vi "UpdatePlugins.vi"(7 "rngInst":refnum<vi>, 8 "Error In Array":errorcluster[](array[cluster]), 10 "Instrument Modules":T1=[{"PluginSelection"=1, "ConfigDialog"=FALSE}, {"PluginSelection"=11, "ConfigDialog"=FALSE}] {"PluginSelection" items=["C37.118 PMU", "C37.118 Sim", "Base PMU", "none", "SiemensDEM0", "AcPwrBase", "Chroma0", "Chroma1", "Chroma2", "NHRDC0", "NHRRGS0", "PPS0"]}, 11 "Current Paths":path[](array[path])) -> (0 "Error Out Array":errorcluster[](array[cluster]), 3 "Current Paths":string[](array[string])=["..\\UserFiles\\Plugins\\AcPwr", "..\\UserFiles\\Plugins\\Sensor"], 4 "PluginTypes":string[](array[string]))   [LabVIEW 2018]
doc: "This VI allows the user to update which Plugins can be selected at the application layer by modifing the location(s) of the INI file(s)."
uses:
  Framework/InstrumentModulesControl.ctl
  <userlib>/NIST/NISTErrorLib/NISTErrorLib.lvlib
panel:
  in  "Save Button":bool
  in  "Update Plugins":bool
  in  "Instrument Modules":T1=[{"PluginSelection"=4, "ConfigDialog"=FALSE}] {"PluginSelection" items=["C37.118 PMU", "C37.118 Sim", "Base PMU", "none", "SiemensDEM0", "AcPwrBase", "Chroma0", "Chroma1", "Chroma2", "NHRDC0", "NHRRGS0", "PPS0"]}
  in  "Cancel  Button":bool
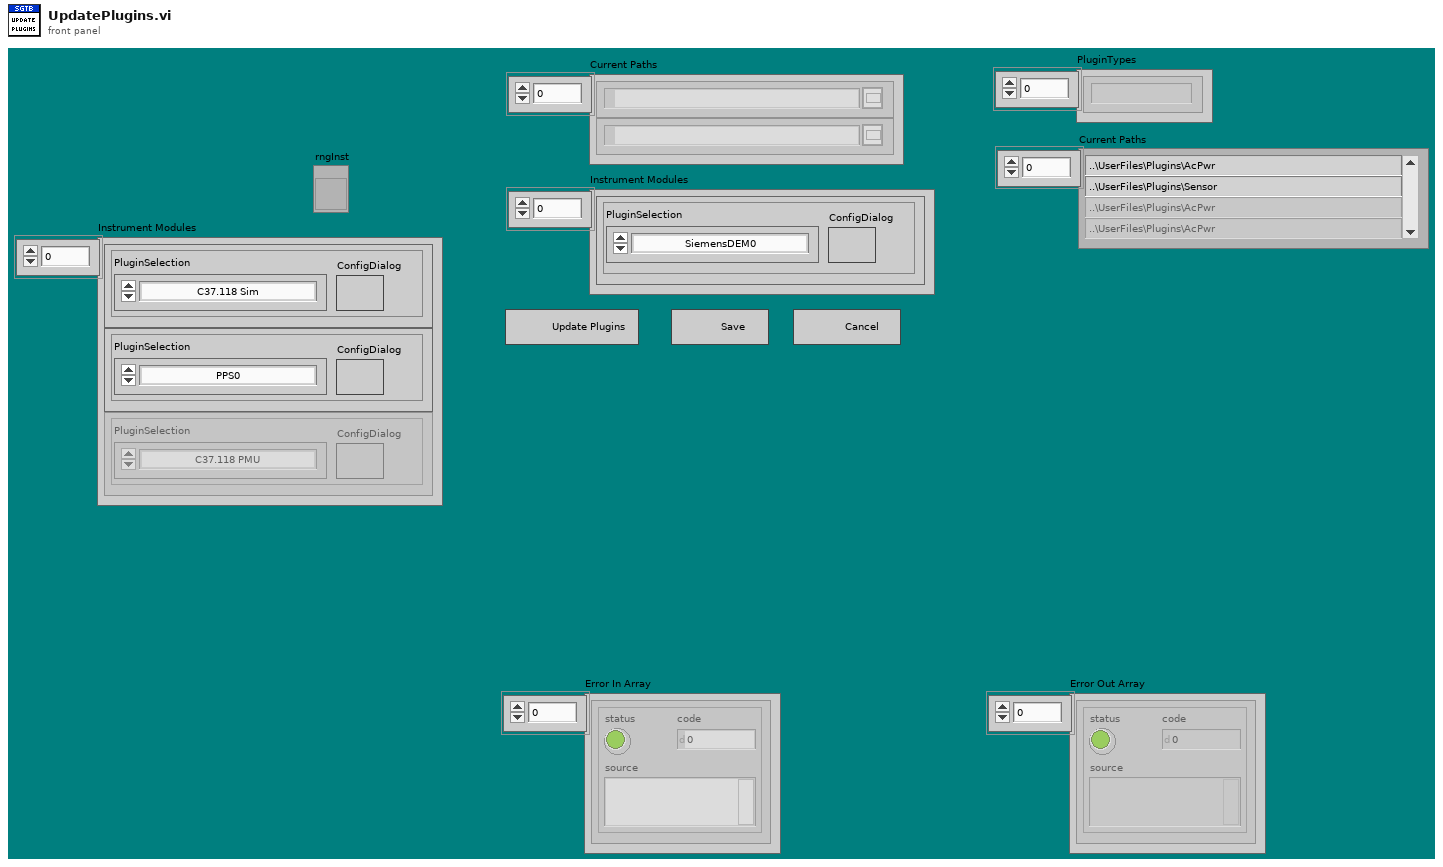
[diagram p1: front panel]
types:
  T1 = typedef "InstrumentModulesControl.ctl" = cluster{"PluginSelection":u16, "ConfigDialog":bool}[]
  T2 = enum32{"Invalid", "Standard", "Closed", "Hidden", "Minimized", "Maximized"}
  T3 = enum32{"Invalid", "Default", "Floating", "Floating/Auto-Hide", "Modal"}
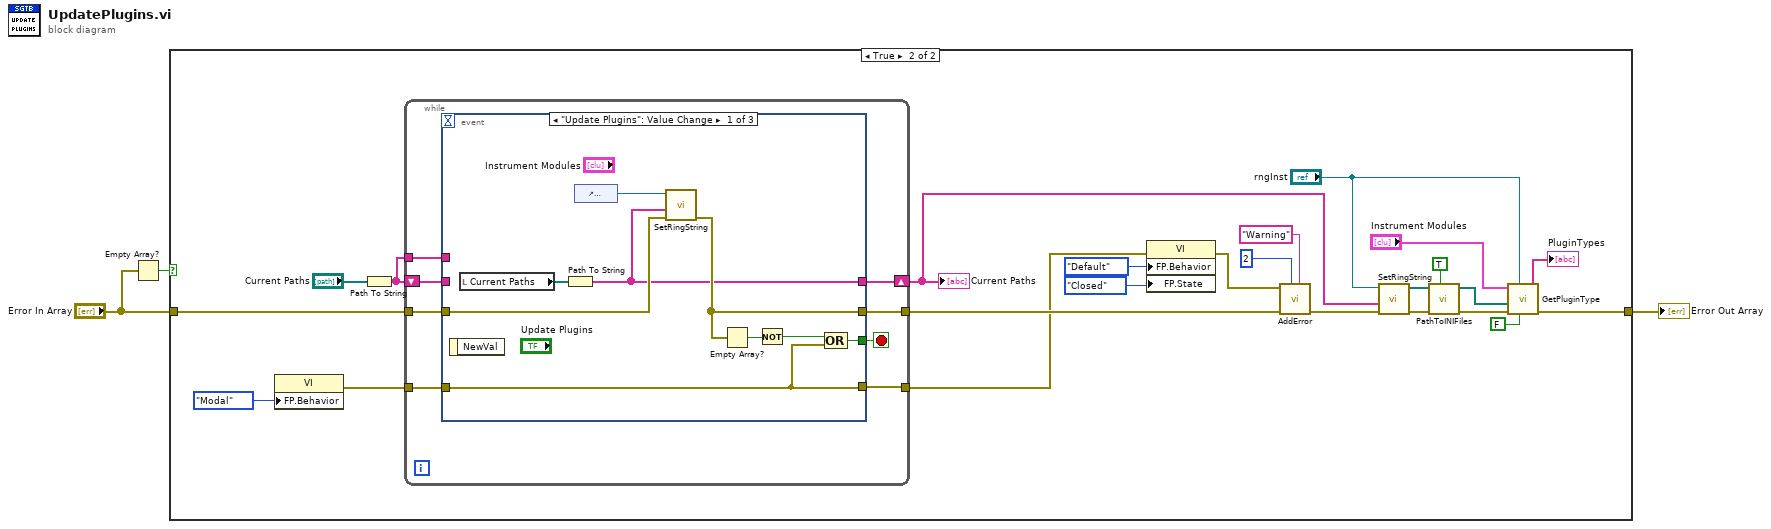
[diagram p0: block diagram]
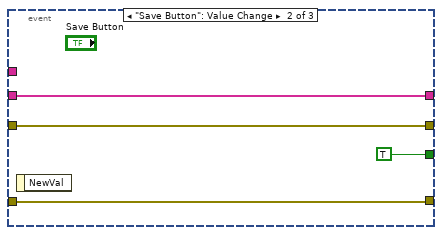
[diagram p3: hidden frame]
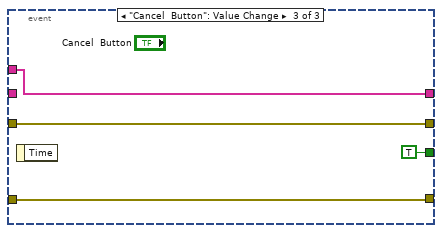
[diagram p4: hidden frame]
diagram:
  n1 = Empty Array?(array="Error In Array") -> (empty?=w2:bool)
  n2 = case shown="True" w2 {
    tunnel: "Error In Array" -> [w4 w27]
    tunnel: [w4 w9] -> w1
    frame False {
    }
    frame True {
      n3 = property class="VI"("FP.Behavior"=T3."Modal" ("Front Panel Window:Behavior")) -> (error out=w25:errorcluster)  [unwired: 2 in, 1 out]
      n4 = Path To String(path="Current Paths") -> (string=w5:string[])
      n5 = while {
        tunnel: w27 -> [w35]
        tunnel: [w33] -> w20
        tunnel: w25 -> [w32]
        tunnel: [w29] -> w18
        shift-right: [w30] -> w8
        shift-left: w5 -> [w31]
        tunnel: w5 -> [w28]
        stop <- w34 stop-if-true
        n6 = event shown="[0] \"Update Plugins\": Value Change" {
          selector: _ -> [_ _ _]
          dyn-events: _ -> [_ _ _]
          timeout: _ -> [_ _ _]
          tunnel: w35 -> [w44 w47 w51]
          tunnel: [w41 TRUE TRUE] -> w34
          tunnel: [w40 w47 w51] -> w33
          tunnel: w32 -> [w38 w45 w50]
          tunnel: w31 -> [_ w46 _]
          tunnel: [w36 w46 w52] -> w30
          tunnel: [w38 w45 w50] -> w29
          tunnel: w28 -> [_ _ w52]
          event "Update Plugins": Value Change {
            n7 = event-data() -> ()  [unwired: 1 in, 1 out]
            n8 = local read "Current Paths"() -> (w37:path[])
            n9 = Path To String(path=w37) -> (string=w36:string[])
            n10 = control-ref of="PluginSelection"() -> (w39:refnum<vi>)
            n11 = call "SetRingString.vi"("ErrorArray In"=w44, "RelativePathToINIFiles"=w36, "Ring in"=w39) -> ("ErrorArray Out out"=w40:errorcluster[])  [unwired: 7 in, 1 out]
            n12 = Empty Array?(array=w40) -> (empty?=w43:bool)
            n13 = Not(x=w43) -> (.not. x?=w42:bool)
            n14 = Compound Arithmetic op=OR(w42, w38) -> (w41:bool)
          }
          event "Save Button": Value Change {
            n15 = event-data() -> ()  [unwired: 1 in, 1 out]
          }
          event "Cancel  Button": Value Change {
            n16 = event-data() -> ()  [unwired: 1 in, 1 out]
          }
        }
      }
      "Current Paths" <- w8
      n17 = property class="VI"(error in=w18, "FP.Behavior"=T3."Default" ("Front Panel Window:Behavior"), "FP.State"=T2."Closed" ("Front Panel Window:State")) -> (error out=w21:errorcluster)  [unwired: 1 in, 1 out]
      n18 = call <userlib>:"AddError.vi"("Severity"="Warning", "Priority"=u8 2, "ErrorArray"=w20, "error in (no error)"=w21) -> ("ErrorArray"=w10:errorcluster[])  [unwired: 6 in, 1 out]
      n19 = call "SetRingString.vi"("ErrorArray In"=w10, "RelativePathToINIFiles"=w8, "Ring in"="rngInst") -> ("ErrorArray Out out"=w13:errorcluster[], "IniFilePaths"=w14:path[])  [unwired: 7 in]
      n20 = call "PathToINIFiles.vi"("Boolean"=TRUE, "IniFilePaths In"=w14) -> ("IniFilePaths Out"=w15:path[])  [unwired: 9 in]
      n21 = call "GetPluginType.vi"("Compare? (F)"=FALSE, "reference"="rngInst", "ErrorArray In"=w13, "INIFilePaths"=w15, "Instrument Modules In New"="Instrument Modules") -> ("ErrorArray Out"=w9:errorcluster[], "PluginTypes"=→"PluginTypes":string[])  [unwired: 2 in, 3 out]
    }
  }
  "Error Out Array" <- w1
